vi "Field Update.vi"(8 "error in (no error)":errorcluster, 10 "Field Record":T2={"ixField"=0, "iSequenceOrder"=0, "sxFieldId"="", "sxSequenceId"="", "sDisplayName"="", "sValue"="", "sUnits"="", "nDataType"=enum."timestamp", "nNextItem"=enum."Reset", "fSystem"=FALSE, "fSystemValue"=FALSE, "fRequired"=FALSE, "fSetAtTest"=FALSE, "fTestField"=FALSE, "fDeleted"=FALSE, "fIndexed"=FALSE, "fFreeList"=FALSE} caption="Field Information", 11 "Connection Refnum":T1) -> (0 "error out":errorcluster, 3 "Connection Refnum":T1)   [LabVIEW 2011]
uses:
  Field Record.ctl
  Field DataTypes.ctl
  Field NextItem.ctl
  Summitek EXT/ODBC/SQL Controls/Connection Refnum.ctl
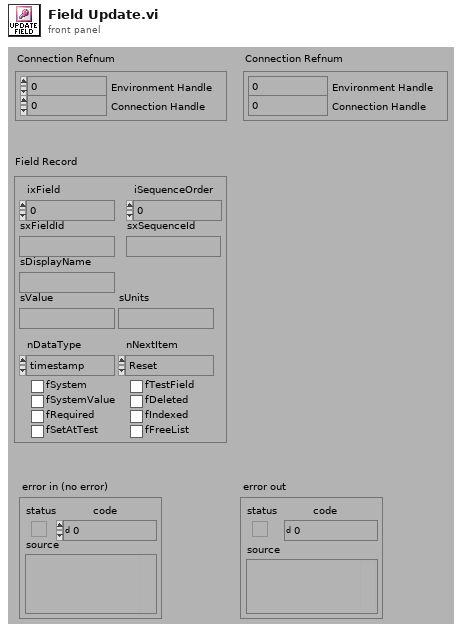
[diagram p1: front panel]
types:
  T1 = typedef "Connection Refnum.ctl" = cluster{"Environment Handle":i32, "Connection Handle":i32}
  T2 = typedef "Field Record.ctl" = cluster{"ixField":i32, "iSequenceOrder":i32, "sxFieldId":string, "sxSequenceId":string, "sDisplayName":string, "sValue":string, "sUnits":string, "nDataType":T3, "nNextItem":T4, "fSystem":bool, "fSystemValue":bool, "fRequired":bool, "fSetAtTest":bool, "fTestField":bool, "fDeleted":bool, "fIndexed":bool, "fFreeList":bool}
  T3 = typedef "Field DataTypes.ctl" = enum32{"text", "numeric", "list", "timestamp", "boolean"}
  T4 = typedef "Field NextItem.ctl" = enum32{"Reset", "Retain", "Auto-Increment"}
  T5 = typedef "Statement Refnum.ctl" = cluster{"Statement Handle":i32, "Parameter Number":u16}
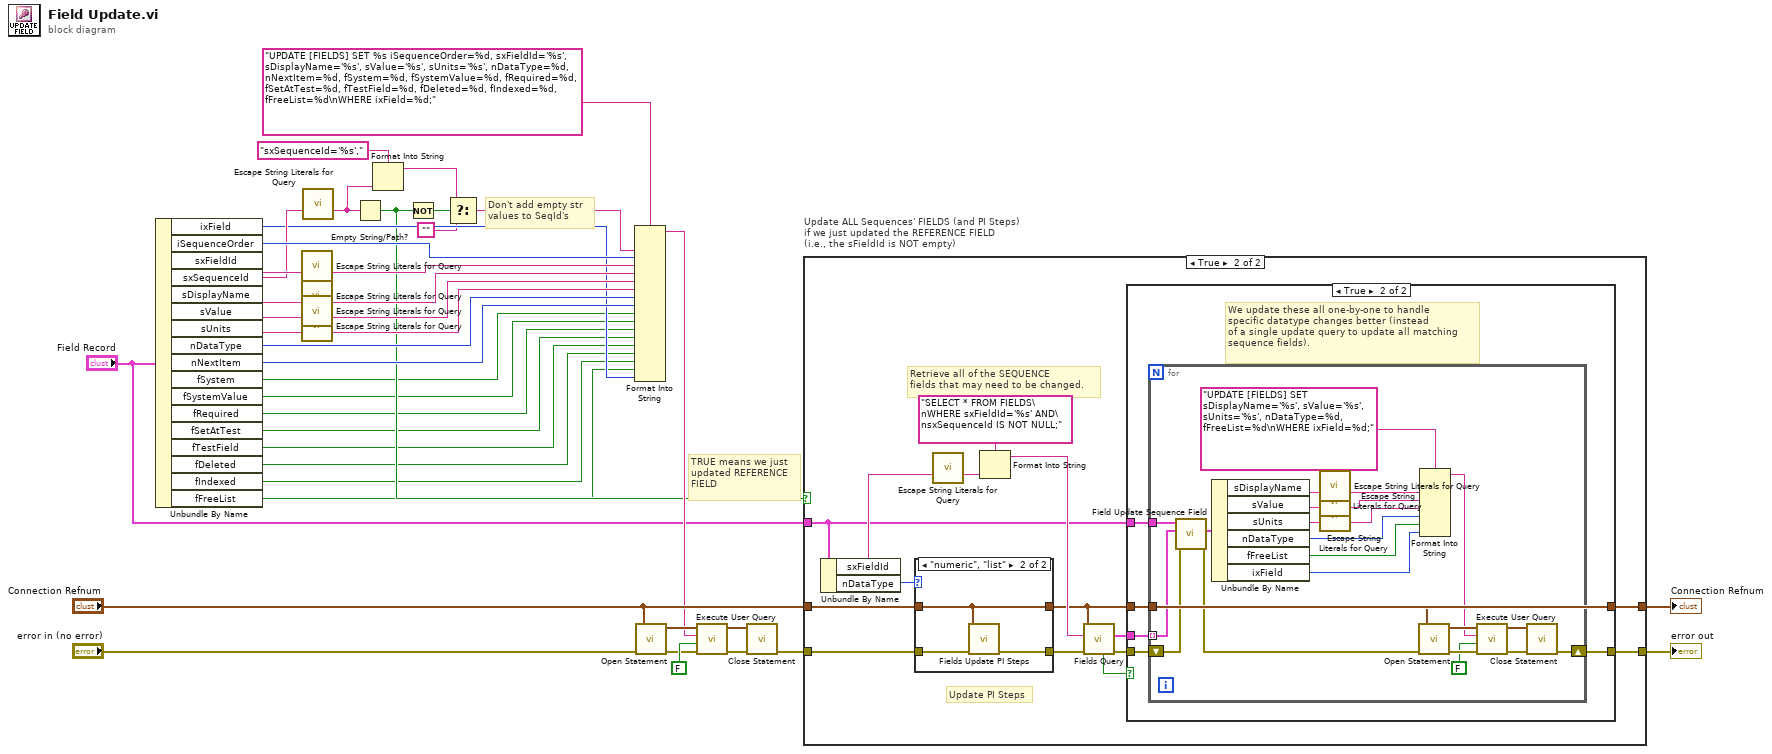
[diagram p0: block diagram]
diagram:
  # "TRUE means we just\nupdated REFERENCE\nFIELD"
  # "Don't add empty str\nvalues to SeqId's"
  n1 = Unbundle By Name("Field Record") -> ("ixField"=w18:i32, "iSequenceOrder"=w31:i32, "sxFieldId"=w30:string, "sxSequenceId"=w29:string, "sDisplayName"=w28:string, "sValue"=w27:string, "sUnits"=w25:string, "nDataType"=w23:T3, "nNextItem"=w22:T4, "fSystem"=w11:bool, "fSystemValue"=w10:bool, "fRequired"=w9:bool, "fSetAtTest"=w8:bool, "fTestField"=w7:bool, "fDeleted"=w6:bool, "fIndexed"=w4:bool, "fFreeList"=w3:bool)
  n2 = call "Escape String Literals for Query.vi"("String"=w30) -> ("escaped String"=w19:string)  [unwired: 1 in, 13 out]
  n3 = call "Escape String Literals for Query.vi"("String"=w28) -> ("escaped String"=w20:string)  [unwired: 1 in, 13 out]
  n4 = call "Escape String Literals for Query.vi"("String"=w27) -> ("escaped String"=w26:string)  [unwired: 1 in, 13 out]
  n5 = call "Escape String Literals for Query.vi"("String"=w25) -> ("escaped String"=w24:string)  [unwired: 1 in, 13 out]
  n6 = call "Escape String Literals for Query.vi"("String"=w29) -> ("escaped String"=w16:string)  [unwired: 1 in, 13 out]
  n7 = Empty String/Path?(string/path=w16) -> (empty?=w15:bool)
  n8 = Format Into String(format string="sxSequenceId='%s'," ("User Query"), w16) -> (resulting string=w13:string)  [unwired: 2 in, 1 out]
  n9 = Not(x=w15) -> (.not. x?=w14:bool)
  n10 = Select(t=w13, s=w14, f="") -> (s? t:f=w5:string)
  n11 = Format Into String(format string="UPDATE [FIELDS] SET %s iSequenceOrder=%d, sxFieldId='%s', sDisplayName='%s', sValue='%s', sUnits='%s', nDataType=%d, nNextItem=%d, fSystem=%d, fSystemValue=%d, fRequired=%d, fSetAtTest=%d, fTestField=%d, fDeleted=%d, fIndexed=%d, fFreeList=%d\nWHERE ixField=%d;" ("User Query"), w5, w31, w19, w20, w26, w24, w23, w22, w11, w10, w9, w8, w7, w6, w4, w3, w18) -> (resulting string=w21:string)  [unwired: 2 in, 1 out]
  n12 = call "Open Statement.vi"("error in (no error)"="error in (no error)", "Connection Refnum"="Connection Refnum") -> ("error out"=w38:errorcluster, "Statement Refnum"=w37:T5)  [unwired: 4 out]
  n13 = call "Execute User Query.vi"("error in (no error)"=w38, "Return Data? (f)"=FALSE, "User Query"=w21, "Statement Refnum"=w37) -> ("error out"=w40:errorcluster, "Statement Refnum"=w39:T5)  [unwired: 2 out]
  n14 = call "Close Statement.vi"("error in (no error)"=w40, "Statement Refnum"=w39) -> ("error out"=w36:errorcluster)  [unwired: 5 out]
  n15 = case "Update ALL Sequences' FIELDS (and PI Steps)\nif we just updated the REFERENCE FIELD\n(i.e., the sFieldId is NOT empty)" shown="True" w15 {
    tunnel: w36 -> [w42 w58]
    tunnel: "Connection Refnum" -> [w43 w57]
    tunnel: [w43 w48] -> w35
    tunnel: [w42 w46] -> w34
    tunnel: "Field Record" -> [_ w44]
    frame False {
      # "FALSE CASE MEANS WE UPDATED A SEQUENCE FIELD ONLY\n\nNo other updates necessary..."
    }
    frame True {
      # "Retrieve all of the SEQUENCE\nfields that may need to be changed."
      # "Update PI Steps"
      n16 = Unbundle By Name(w44) -> ("sxFieldId"=w55:string, "nDataType"=w56:T3)
      n17 = case shown="\"numeric\", \"list\"" w56 {
        tunnel: w58 -> [w89 w93]
        tunnel: w57 -> [w90 w91]
        tunnel: [w89 w92] -> w51
        tunnel: [w90 w91] -> w49
        frame Default {
        }
        frame "numeric", "list" {
          n18 = call "Fields Update PI Steps.vi"("error in (no error)"=w93, "Connection Refnum"=w91) -> ("error out"=w92:errorcluster)  [unwired: 9 out]
        }
      }
      n19 = call "Escape String Literals for Query.vi"("String"=w55) -> ("escaped String"=w52:string)  [unwired: 1 in, 13 out]
      n20 = Format Into String(format string="SELECT * FROM FIELDS\nWHERE sxFieldId='%s' AND\nsxSequenceId IS NOT NULL;" ("Query Name"), w52) -> (resulting string=w53:string)  [unwired: 2 in, 1 out]
      n21 = call "Fields Query.vi"("error in (no error)"=w51, "Query"=w53, "Connection Refnum"=w49) -> ("error out"=w47:errorcluster, "Fields"=w45:T2[], "Data Present?"=w50:bool)  [unwired: 1 in, 5 out]
      n22 = case shown="True" w50 {
        tunnel: w49 -> [w60 w65]
        tunnel: [w60 w65] -> w48
        tunnel: w47 -> [w59 w63]
        tunnel: [w59 w64] -> w46
        tunnel: w45 -> [_ w62]
        tunnel: w44 -> [_ w61]
        frame False {
        }
        frame True {
          # "We update these all one-by-one to handle\nspecific datatype changes better (instead\nof a single update query to update all matching\nsequence fields)."
          n23 = for {
            tunnel: w65 -> [w88]
            shift-right: [w82] -> w64
            shift-left: w63 -> [w79]
            tunnel: w62 -> [w81] mode=indexing
            tunnel: w61 -> [w80]
            n24 = call "Field Update Sequence Field.vi"("error in (no error)"=w79, "Original Sequence Field Record"=w81, "New Sequence Field Record"=w80) -> ("error out"=w78:errorcluster, "Updated Field Record"=w75:T2)  [unwired: 7 out]
            n25 = Unbundle By Name(w75) -> ("sDisplayName"=w73:string, "sValue"=w72:string, "sUnits"=w71:string, "nDataType"=w68:T3, "fFreeList"=w67:bool, "ixField"=w66:i32)
            n26 = call "Escape String Literals for Query.vi"("String"=w73) -> ("escaped String"=w74:string)  [unwired: 1 in, 13 out]
            n27 = call "Escape String Literals for Query.vi"("String"=w72) -> ("escaped String"=w70:string)  [unwired: 1 in, 13 out]
            n28 = call "Escape String Literals for Query.vi"("String"=w71) -> ("escaped String"=w69:string)  [unwired: 1 in, 13 out]
            n29 = call "Open Statement.vi"("error in (no error)"=w78, "Connection Refnum"=w88) -> ("error out"=w86:errorcluster, "Statement Refnum"=w87:T5)  [unwired: 4 out]
            n30 = Format Into String(format string="UPDATE [FIELDS] SET sDisplayName='%s', sValue='%s', sUnits='%s', nDataType=%d, fFreeList=%d\nWHERE ixField=%d;" ("User Query"), w74, w70, w69, w68, w67, w66) -> (resulting string=w77:string)  [unwired: 2 in, 1 out]
            n31 = call "Execute User Query.vi"("error in (no error)"=w86, "Return Data? (f)"=FALSE, "User Query"=w77, "Statement Refnum"=w87) -> ("error out"=w84:errorcluster, "Statement Refnum"=w85:T5)  [unwired: 2 out]
            n32 = call "Close Statement.vi"("error in (no error)"=w84, "Statement Refnum"=w85) -> ("error out"=w82:errorcluster)  [unwired: 5 out]
          }
        }
      }
    }
  }
  "error out" <- w34
  "Connection Refnum" <- w35
